vi "Module Cleanup.vi"(8 "error in (no error)":errorcluster, 11 "ValveSimModule in":refnum<class "ValveSimModule.lvclass">) -> (0 "error out":errorcluster, 3 "ValveSimModule out":refnum<class "ValveSimModule.lvclass">)   [LabVIEW 2020, in "VolatusScratch.lvlib" / "ValveSimModule.lvclass"]
uses:
  ValveSimModule.lvclass
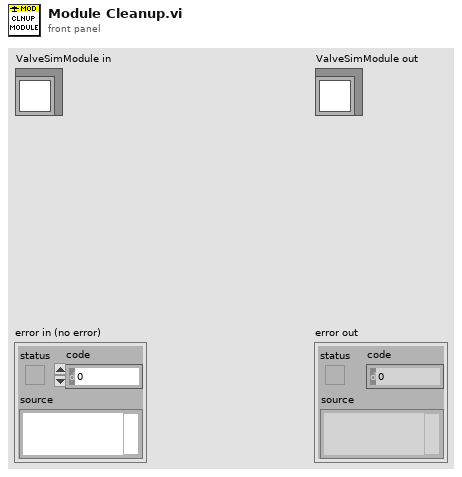
[diagram p1: front panel]
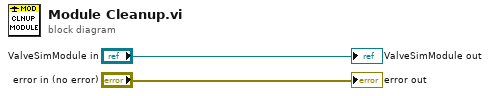
[diagram p0: block diagram]
diagram:
  "error out" <- "error in (no error)"
  "ValveSimModule out" <- "ValveSimModule in"
